vi "GetLoopShiftRegisters.vi"(5 "Loop in":refnum<class "Loop.lvclass">, 6 "error in":errorcluster, 9 "VI Interpreter in":refnum<class "VI Interpreter.lvclass">) -> (0 "error out":errorcluster, 3 "VI Interpreter out":refnum<class "VI Interpreter.lvclass">, 4 "Loop out":refnum<class "Loop.lvclass">)   [LabVIEW 2014, in "VI Interpreter.lvclass"]
uses:
  VI Interpreter.lvclass
  Loop/Loop.lvclass
  ShiftRegister/ShiftRegister.lvclass
  ShiftRegister/ShiftRegister.lvclass/ShiftRegister.ctl
  Loop/Loop.lvclass/Loop.ctl
  RightShiftRegister/RightShiftRegister.lvclass
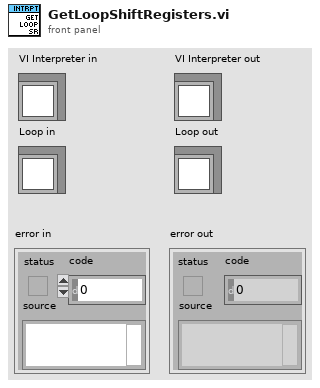
[diagram p1: front panel]
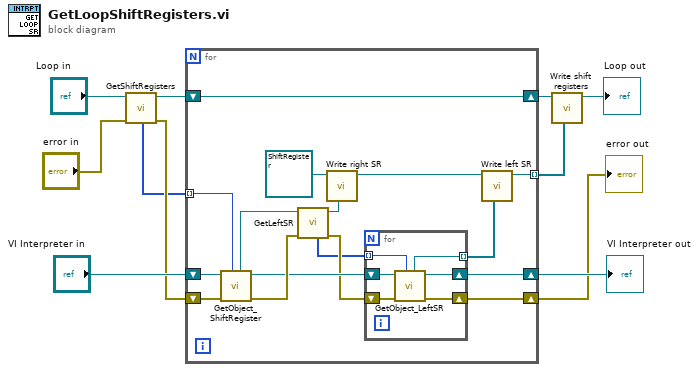
[diagram p0: block diagram]
diagram:
  n1 = call "GetShiftRegisters.vi"("error in"="error in", "Loop in"="Loop in") -> ("error out"=w6:errorcluster, "Loop out"=w2:refnum<class "Loop.lvclass">, "shift registers"=w5:i32[])  [unwired: 5 in]
  n2 = for {
    shift-right: [w20] -> w10
    shift-left: "VI Interpreter in" -> [w27]
    shift-right: [w21] -> w9
    shift-left: w6 -> [w26]
    tunnel: w5 -> [w25] mode=indexing
    tunnel: [w15] -> w3 mode=indexing
    shift-right: [w12] -> w1
    shift-left: w2 -> [w12]
    n3 = call "GetObject_ShiftRegister.vi"("UID"=w25, "error in"=w26, "VI Interpreter in"=w27) -> ("error out"=w23:errorcluster, "VI Interpreter out"=w22:refnum<class "VI Interpreter.lvclass">, "SR"=w24:refnum<class "RightShiftRegister.lvclass">)  [unwired: 3 in, 1 out]
    n4 = call "GetLeftSR.vi"("error in"=w23, "RightShiftRegister in"=w24) -> ("error out"=w19:errorcluster, "RightShiftRegister out"=w13:refnum<class "RightShiftRegister.lvclass">, "left SR"=w18:i32[])  [unwired: 7 in]
    n5 = call "Write right SR.vi"("right SR"=w13, "ShiftRegister in"=refnum<class "ShiftRegister.lvclass"> refnum ("ShiftRegister.lvclass")) -> ("ShiftRegister out"=w14:refnum<class "ShiftRegister.lvclass">)  [unwired: 7 in]
    n6 = for {
      shift-right: [w30] -> w20
      shift-left: w22 -> [w33]
      shift-right: [w31] -> w21
      shift-left: w19 -> [w32]
      tunnel: w18 -> [w29] mode=indexing
      tunnel: [w28] -> w16 mode=indexing
      n7 = call "GetObject_LeftSR.vi"("UID"=w29, "error in"=w32, "VI Interpreter in"=w33) -> ("error out"=w31:errorcluster, "VI Interpreter out"=w30:refnum<class "VI Interpreter.lvclass">, "SR"=w28:refnum<class "LeftShiftRegister.lvclass">)  [unwired: 3 in, 1 out]
    }
    n8 = call "Write left SR.vi"("left SR"=w16, "ShiftRegister in"=w14) -> ("ShiftRegister out"=w15:refnum<class "ShiftRegister.lvclass">)  [unwired: 7 in]
  }
  "error out" <- w9
  "VI Interpreter out" <- w10
  n9 = call "Write shift registers.vi"("shift registers"=w3, "Loop in"=w1) -> ("Loop out"=→"Loop out":refnum<class "Loop.lvclass">)  [unwired: 7 in]
